vi "Write N Registers.vi"(8 "Error In":errorcluster, 9 "Data":u8[](array[numeric]), 10 "Register Addresses":u8[](array[numeric]), 11 "Adept Config":T1) -> (0 "Error Out":errorcluster, 3 "Adept Config":T1)   [LabVIEW 2011, in "LVH-Adept.lvlib"]
uses:
  LVH-Adept.lvlib
  Private/Type Defs/Device Config.ctl
  Private/Type Defs/Status.ctl
  Private/DEPP/DEPP.lvlib
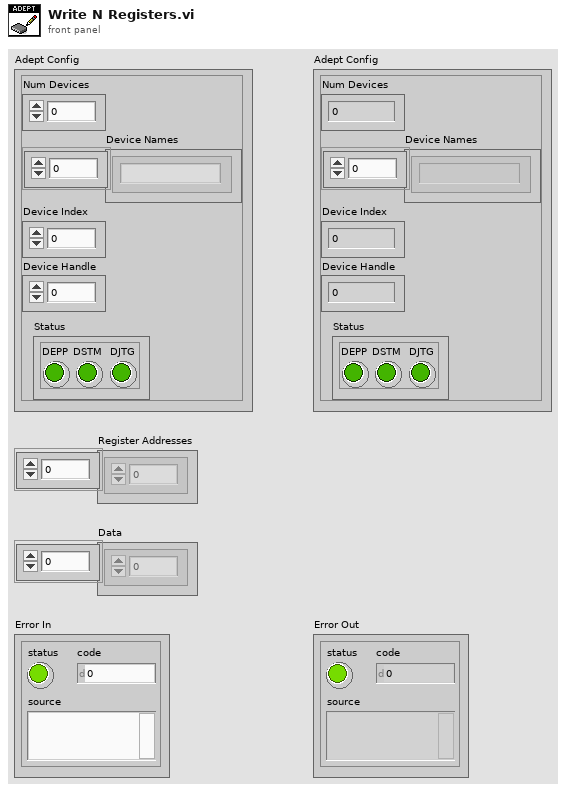
[diagram p1: front panel]
types:
  T1 = typedef "LVH-Adept.lvlib/Device Config.ctl" = cluster{"Num Devices":i32, "Device Names":string[], "Device Index":u16, "Device Handle":u32, "Status":T2}
  T2 = typedef "LVH-Adept.lvlib/Status.ctl" = cluster{"DEPP":bool, "DSTM":bool, "DJTG":bool}
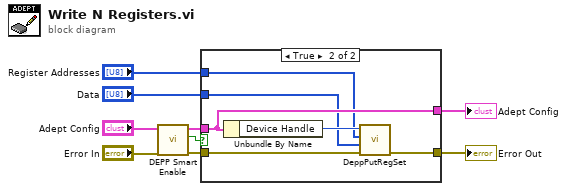
[diagram p0: block diagram]
diagram:
  n1 = call "DEPP Smart Enable.vi"("Error In"="Error In", "Adept Config"="Adept Config") -> ("Error Out"=w7:errorcluster, "Success?"=w6:bool, "Adept Config"=w4:T1)  [unwired: 7 in]
  n2 = case shown="True" w6 {
    tunnel: w7 -> [w11 w15]
    tunnel: w4 -> [w10 w17]
    tunnel: "Register Addresses" -> [_ w12]
    tunnel: [w11 w16] -> w5
    tunnel: [w10 w17] -> w3
    tunnel: "Data" -> [_ w13]
    frame False {
    }
    frame True {
      n3 = Unbundle By Name(w17) -> ("Device Handle"=w14:u32)
      n4 = call "DeppPutRegSet.vi"("Error In"=w15, "Data"=w13, "Addresses"=w12, "Device Handle"=w14) -> ("Error Out"=w16:errorcluster)  [unwired: 6 in, 1 out]
    }
  }
  "Error Out" <- w5
  "Adept Config" <- w3
